vi "CTI_AOTF-Init.vi"(8 "error in":errorcluster) -> (0 "error out":errorcluster, 3 "Config Out":string[](array[string]))   [LabVIEW 2013]
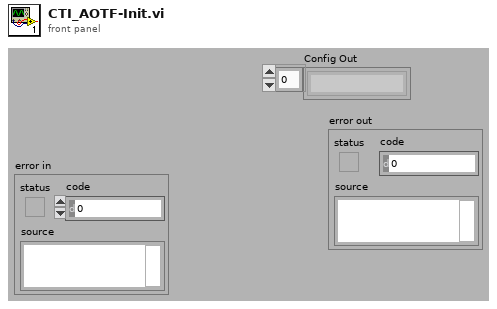
[diagram p1: front panel]
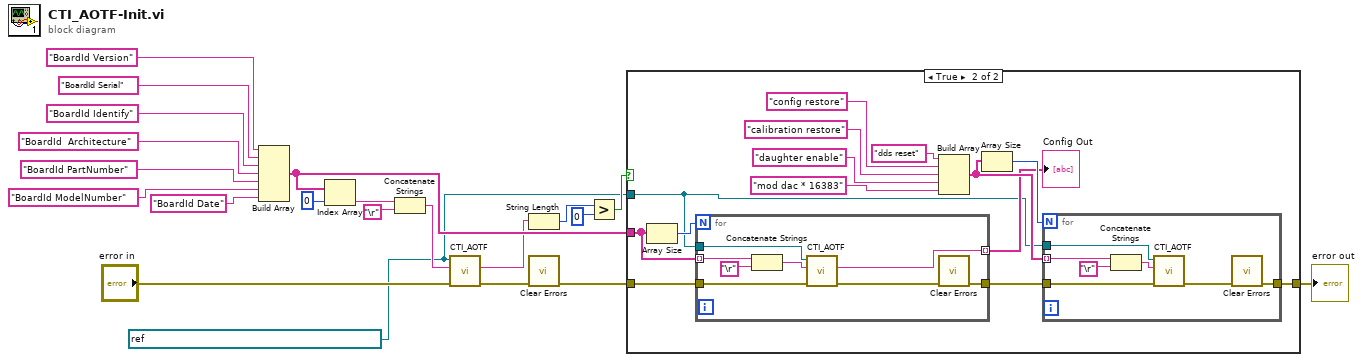
[diagram p0: block diagram]
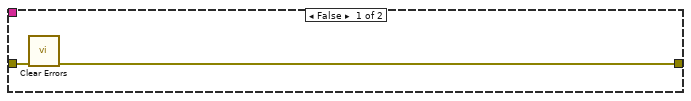
[diagram p2: hidden frame]
diagram:
  w1 = refnum<visa-resource-name> "USB0::0x16C7::0x0001::NI-VISA-20001::RAW" ("VISA resource name 2")
  n1 = Build Array("BoardId Version" ("string"), "BoardId Serial" ("string"), "BoardId Identify" ("string"), "BoardId  Architecture" ("string"), "BoardId PartNumber" ("string"), "BoardId ModelNumber" ("element"), "BoardId Date" ("element")) -> (w12:string[])
  n2 = Index Array(array=w12, index=0) -> (element=w10:string)
  n3 = Concatenate Strings(w10, "\r") -> (w5:string)
  n4 = call "CTI_AOTF.vi"("error in"="error in", "String"=w5, "VISA resource name 2"=w1) -> ("error out"=w3:errorcluster, "read buffer"=w4:string)  [unwired: 7 in]
  n5 = String Length(string=w4) -> (length=w8:i32)
  n6 = call <vilib>:"Clear Errors.vi"("error in (no error)"=w3) -> ("error out"=w9:errorcluster)  [unwired: 6 out]
  n7 = Greater?(x=w8, y=0) -> (0:w6:bool)
  n8 = case shown="True" w6 {
    tunnel: [w23 w24] -> w21
    tunnel: w12 -> [_ w27]
    tunnel: w1 -> [_ w25]
    tunnel: w9 -> [w22 w26]
    frame False {
      n9 = call <vilib>:"Clear Errors.vi"("error in (no error)"=w22) -> ("error out"=w23:errorcluster)  [unwired: 6 in]
    }
    frame True {
      n10 = Array Size(array=w27) -> (size(s)=w30:i32)
      n11 = for {
        N: w30 -> [_]
        tunnel: [w45] -> w29
        tunnel: w25 -> [w41]
        tunnel: w27 -> [w44] mode=indexing
        tunnel: [w38] -> w28 mode=indexing
        tunnel: w26 -> [w40]
        n12 = Concatenate Strings(w44, "\r") -> (w42:string)
        n13 = call "CTI_AOTF.vi"("error in"=w40, "String"=w42, "VISA resource name 2"=w41) -> ("error out"=w39:errorcluster, "read buffer"=w38:string)  [unwired: 7 in]
        n14 = call <vilib>:"Clear Errors.vi"("error in (no error)"=w39) -> ("error out"=w45:errorcluster)  [unwired: 6 out]
      }
      "Config Out" <- w28
      n15 = Build Array("dds reset" ("string"), "config restore" ("string"), "calibration restore" ("string"), "daughter enable" ("string"), "mod dac * 16383" ("string")) -> (w32:string[])
      n16 = Array Size(array=w32) -> (size(s)=w31:i32)
      n17 = for {
        N: w31 -> [_]
        tunnel: [w52] -> w24
        tunnel: w25 -> [w49]
        tunnel: w32 -> [w51] mode=indexing
        tunnel: w29 -> [w47]
        n18 = Concatenate Strings(w51, "\r") -> (w48:string)
        n19 = call "CTI_AOTF.vi"("error in"=w47, "String"=w48, "VISA resource name 2"=w49) -> ("error out"=w46:errorcluster)  [unwired: 7 in, 1 out]
        n20 = call <vilib>:"Clear Errors.vi"("error in (no error)"=w46) -> ("error out"=w52:errorcluster)  [unwired: 6 out]
      }
    }
  }
  "error out" <- w21
